vi "Get 8 Neighbors.vi"(9 "column":i32, 10 "row":i32, 11 "cells in":bool[][](array[boolean])) -> (3 "cells living":bool[](array[boolean]))   [LabVIEW 2021, in "Game of Life.lvlib"]
uses:
  Game of Life.lvlib
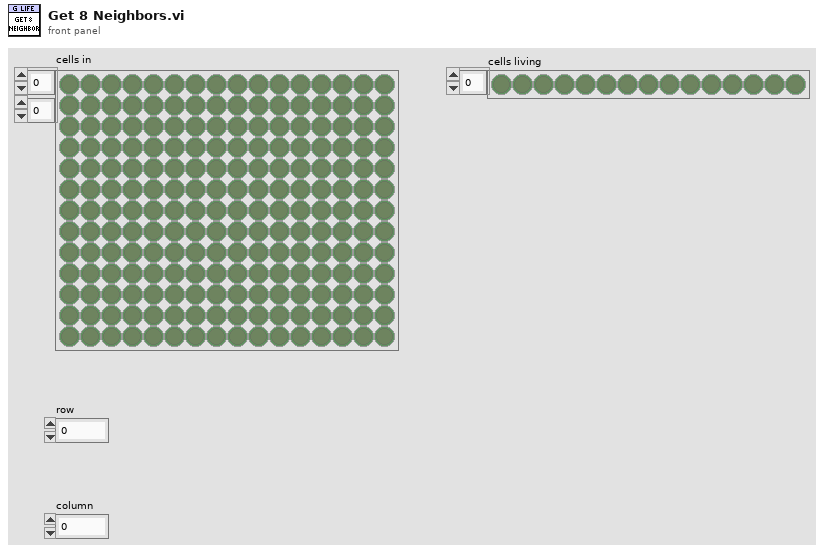
[diagram p1: front panel]
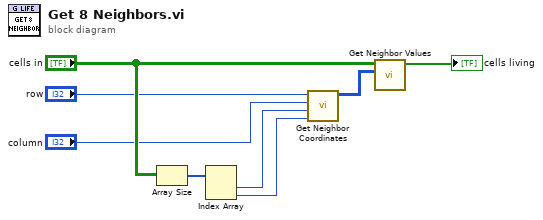
[diagram p0: block diagram]
diagram:
  n1 = Array Size(array="cells in") -> (size(s)=w6:i32[])
  n2 = Index Array(array=w6) -> (element #1=w3:i32, element #2=w2:i32)  [unwired: 2 in]
  n3 = call "Get Neighbor Coordinates.vi"("# cols"=w2, "# rows"=w3, "column"="column", "row"="row") -> ("neighbor coordinates"=w1:i32[][])  [unwired: 7 in]
  n4 = call "Get Neighbor Values.vi"("neighbor coordinates"=w1, "cells in"="cells in") -> ("cells living"=→"cells living":bool[])  [unwired: 9 in]
